vi "Drive Core.vi"(0 "A Encoder BL":string="My Motor RefNum", 1 "Rotational Motor FR":string="My Motor RefNum", 2 "Rotational Motor FL":string="My Motor RefNum", 3 "Rotational Motor BR":string="My Motor RefNum", 4 "Rotational Motor BL":string="My Motor RefNum", 5 "Drive Motor FR":string="My Motor RefNum", 6 "A Encoder BR":string="My Motor RefNum", 7 "Drive Motor FL":string="My Motor RefNum", 8 "A Encoder FL":string="My Motor RefNum", 9 "Drive Motor BR":string="My Motor RefNum", 10 "A Encoder FR":string="My Motor RefNum", 11 "Drive Motor BL":string="My Motor RefNum") -> ()   [LabVIEW 2014]
uses:
  Global Variables.vi
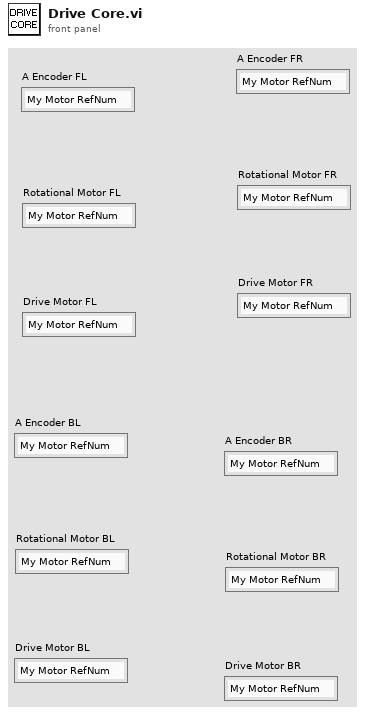
[diagram p1: front panel]
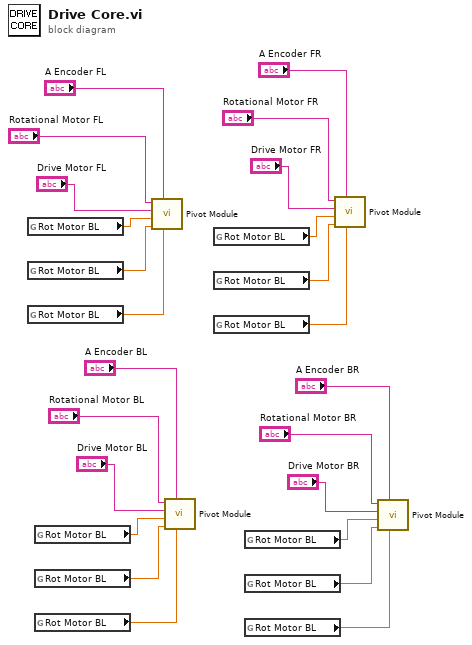
[diagram p0: block diagram]
diagram:
  n1 = global read "Global Variables.vi" "Rot Motor BL"() -> (w12:dbl)
  n2 = global read "Global Variables.vi" "Rot Motor BL"() -> (w11:dbl)
  n3 = global read "Global Variables.vi" "Rot Motor BL"() -> (w10:dbl)
  n4 = global read "Global Variables.vi" "Rot Motor BL"() -> (w6:dbl)
  n5 = global read "Global Variables.vi" "Rot Motor BL"() -> (w5:dbl)
  n6 = global read "Global Variables.vi" "Rot Motor BL"() -> (w4:dbl)
  n7 = call "Pivot Module.vi"("Calibration Angle"=w10, "Encoder Refnum"="A Encoder FL", "Motor Speed"=w11, "Motor Angle"=w12, "Drive Motor Refnum"="Drive Motor FL", "Rotational Motor Refnum"="Rotational Motor FL") -> ()  [unwired: 6 in]
  n8 = call "Pivot Module.vi"("Calibration Angle"=w4, "Encoder Refnum"="A Encoder BL", "Motor Speed"=w5, "Motor Angle"=w6, "Drive Motor Refnum"="Drive Motor BL", "Rotational Motor Refnum"="Rotational Motor BL") -> ()  [unwired: 6 in]
  n9 = global read "Global Variables.vi" "Rot Motor BL"() -> (w9:dbl)
  n10 = global read "Global Variables.vi" "Rot Motor BL"() -> (w8:dbl)
  n11 = global read "Global Variables.vi" "Rot Motor BL"() -> (w7:dbl)
  n12 = global read "Global Variables.vi" "Rot Motor BL"() -> (w3:dbl)
  n13 = global read "Global Variables.vi" "Rot Motor BL"() -> (w2:dbl)
  n14 = global read "Global Variables.vi" "Rot Motor BL"() -> (w1:dbl)
  n15 = call "Pivot Module.vi"("Calibration Angle"=w7, "Encoder Refnum"="A Encoder FR", "Motor Speed"=w8, "Motor Angle"=w9, "Drive Motor Refnum"="Drive Motor FR", "Rotational Motor Refnum"="Rotational Motor FR") -> ()  [unwired: 6 in]
  n16 = call "Pivot Module.vi"("Calibration Angle"=w1, "Encoder Refnum"="A Encoder BR", "Motor Speed"=w2, "Motor Angle"=w3, "Drive Motor Refnum"="Drive Motor BR", "Rotational Motor Refnum"="Rotational Motor BR") -> ()  [unwired: 6 in]
